vi "1WIRE_Write_1_bit.vi"(7 "1-Wire DIO Pin":refnum<k21>="ConnectorA/DIO15", 8 "error in":errorcluster) -> (0 "error out":errorcluster)   [LabVIEW 2014]
doc: "This VI is created by Vincent Claes for FPDA-1 more information on http://pwo.fpga.be\n\nvincent.claes@xios.be\nclaesvincent@gmail.com\n\nhttp://www.linkedin.com/in/vincentclaes"
uses:
  <vilib>/rvi/eio/common/nirviEmuTemplateMethod_errors.vi
  <vilib>/eio/EIOMethodNode/EIOMethodNode.xnode
  <vilib>/eio/EIONode/EIONode.xnode
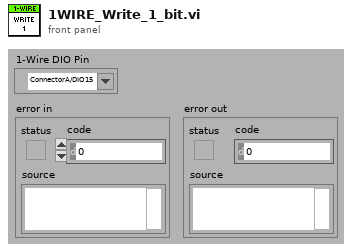
[diagram p1: front panel]
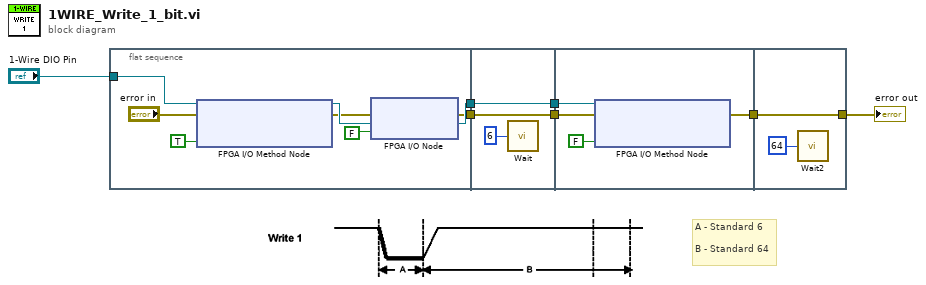
[diagram p0: block diagram]
diagram:
  # "A - Standard 6\n\nB - Standard 64"
  n1 = flat-sequence {
    tunnel: [w13] -> w7
    tunnel: [w10] -> w4
    tunnel: "1-Wire DIO Pin" -> [w8]
    tunnel: w7 -> [w17]
    tunnel: [w17] -> w6
    tunnel: [w16] -> w5
    tunnel: w4 -> [w16]
    tunnel: w6 -> [w21]
    tunnel: w5 -> [w22]
    tunnel: [w20] -> w2
    tunnel: [w23] -> w3
    tunnel: w2 -> [w23]
    frame #0 {
      n2 = xnode "FPGA I/O Method Node"("error in"="error in", "FPGA I/O In"=w8, "Enable"=TRUE) -> ("error out"=w11:errorcluster, "FPGA I/O Out"=w14:refnum<k21>)
      n3 = xnode "FPGA I/O Node"("error in"=w11, "I/O Item"=FALSE ("FX2_IO1_J1_0"), "FPGA I/O In"=w14) -> ("error out"=w10:errorcluster, "FPGA I/O Out"=w13:refnum<k21>)
    }
    frame #1 {
      n4 = call "Wait"("Count(uSec)"=u32 6) -> ()  [unwired: 1 out]
    }
    frame #2 {
      n5 = xnode "FPGA I/O Method Node"("error in"=w22, "FPGA I/O In"=w21, "Enable"=FALSE) -> ("error out"=w20:errorcluster)  [unwired: 1 out]
    }
    frame #3 {
      n6 = call "Wait2"("Count(uSec)"=u32 64) -> ()  [unwired: 1 out]
    }
  }
  "error out" <- w3
